vi "Save-Recall Setup.vi"(0 "VISA resource name":refnum<visa-resource-name>, 5 "Mode(F:Save)":bool, 7 "Address (0)":u32 max=4, 11 "error in (no error)":errorcluster) -> (4 "VISA resource name out":refnum<visa-resource-name>, 15 "error out":errorcluster)   [LabVIEW 2012, in "Agilent 66XX Series.lvlib"]
doc: "This vi controls the memory functions of the DC power supply. The current system setup can be stored in one of five states (one of four states for the E4356a, 668x and 669x series). These parameters are stored in memory locations 0 - 4 (0 - 3 for the above mentioned models)."
uses:
  Agilent 66XX Series.lvlib
panel:
  # "Recall"
  # "Save"
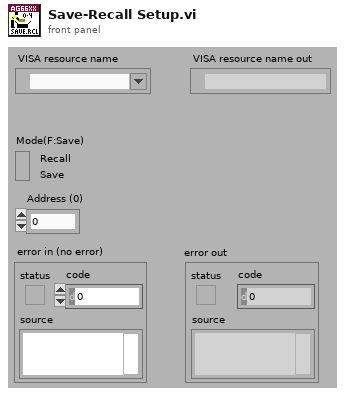
[diagram p1: front panel]
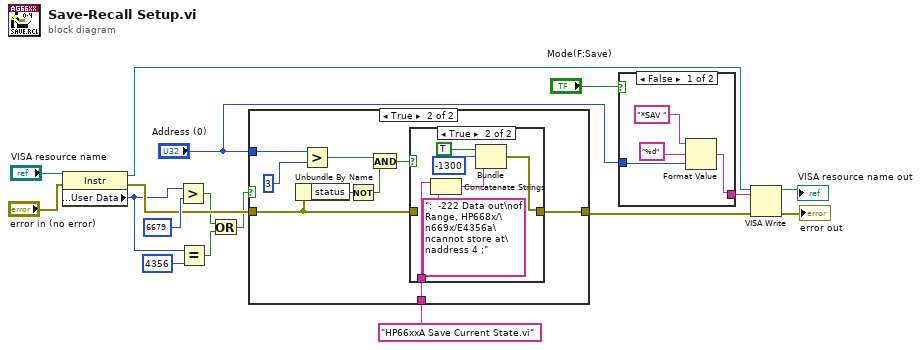
[diagram p0: block diagram]
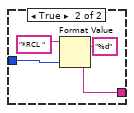
[diagram p2: hidden frame]
diagram:
  n1 = property class="Instr"(reference="VISA resource name", error in="error in (no error)") -> (reference out=w11:refnum<visa-resource-name>, error out=w7:errorcluster, "General Settings:User Data"=w5:u32)
  n2 = Greater?(x=w5, y=u32 6679) -> (0:w3:bool)
  n3 = Equal?(x=w5, y=u32 4356) -> (x = y?=w2:bool)
  n4 = Or(x=w3, y=w2) -> (x .or. y?=w1:bool)
  n5 = case shown="True" w1 {
    tunnel: [w18 w25] -> w15
    tunnel: w7 -> [w18 w23]
    tunnel: "Address (0)" -> [_ w27]
    tunnel: "HP66xxA Save Current State.vi" -> [_ w24]
    frame False {
    }
    frame True {
      n6 = Unbundle By Name(w23) -> ("status"=w22:bool)
      n7 = Greater?(x=w27, y=u32 3) -> (0:w19:bool)
      n8 = Not(x=w22) -> (.not. x?=w20:bool)
      n9 = And(x=w19, y=w20) -> (x .and. y?=w21:bool)
      n10 = case shown="True" w21 {
        tunnel: [w28 w30] -> w25
        tunnel: w23 -> [w28 _]
        tunnel: w24 -> [_ w29]
        frame False {
        }
        frame True {
          n11 = Concatenate Strings(w29, ":  -222 Data out\nof Range, HP668x/\n669x/E4356a\ncannot store at\naddress 4 ;") -> (w31:string)
          n12 = Bundle(TRUE, -1300, w31) -> (w30:errorcluster)  [unwired: 1 in]
        }
      }
    }
  }
  n13 = case shown="False" "Mode(F:Save)" {
    tunnel: [w38 w42] -> w12
    tunnel: "Address (0)" -> [w35 w39]
    frame False {
      n14 = Format Value(string ("")="*SAV ", format string="%d", value (0)=w35) -> (output string=w38:string)
    }
    frame True {
      n15 = Format Value(string ("")="*RCL ", format string="%d", value (0)=w39) -> (output string=w42:string)
    }
  }
  n16 = VISA Write(VISA resource name=w11, write buffer=w12, error in (no error)=w15) -> (VISA resource name out=→"VISA resource name out":refnum<visa-resource-name>, error out=→"error out":errorcluster)  [unwired: 1 out]
